vi "Close.vi"(8 "error in (no error)":errorcluster, 11 "RP Communicator in":refnum<class "RP Communicator VISA.lvclass">) -> (0 "error out":errorcluster, 3 "RP Communicator out":refnum<class "RP Communicator VISA.lvclass">)   [LabVIEW 2019, in "RP Communicator VISA.lvclass"]
uses:
  RP Communicator VISA.lvclass
  RP Command.ctl
  RP Communicator VISA.lvclass/RP Communicator VISA.ctl
  RP Write Command VISA.vi
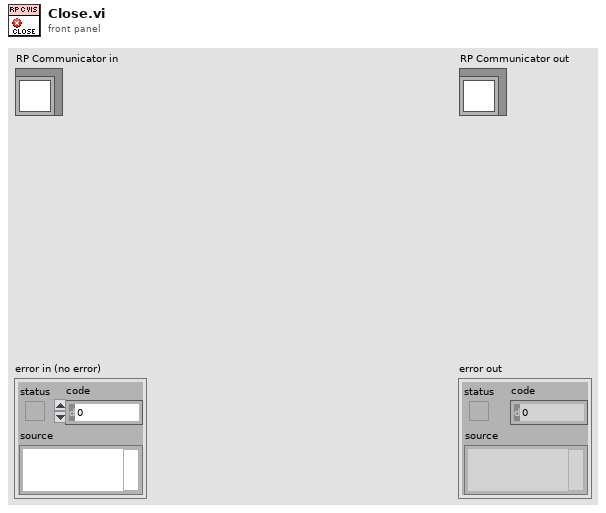
[diagram p1: front panel]
types:
  T1 = typedef "RP Command.ctl" = enum16{"Reset", "Read IDN", "Stop server", "Get status", "Get temperature", "Connect client", "Arm", "Software trigger", "Get whole buffer", "Get chunk", "System call", "Get config", "Set config", "Recieve data", "Recieve Calibartion", "Transmit data"}
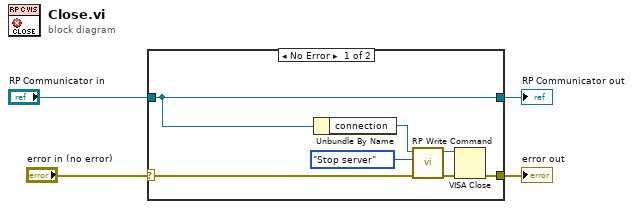
[diagram p0: block diagram]
diagram:
  n1 = case shown="No Error" "error in (no error)" {
    selector: "error in (no error)" -> [w8 w13]
    tunnel: [w5 w13] -> w3
    tunnel: [w11 w12] -> w1
    tunnel: "RP Communicator in" -> [w11 w12]
    frame No Error {
      n2 = Unbundle By Name(w11) -> ("connection"=w10:refnum<visa-resource-name>)
      n3 = call-poly "RP Write Command.vi"("Error In"=w8, "Command number"=RP_Command."Stop server", "VISA resource"=w10) -> ("Error Out"=w7:errorcluster, "VISA resource out"=w6:refnum<visa-resource-name>)  [unwired: 6 in, 1 out]
      n4 = VISA Close(VISA resource name=w6, error in (no error)=w7) -> (error out=w5:errorcluster)
    }
    frame Error {
    }
  }
  "error out" <- w3
  "RP Communicator out" <- w1
